vi "Reply.vi"(8 "error in (no error)":errorcluster, 10 "Reply":refnum<class "MSG.lvclass"> caption="Reply (Label superceeded by reply label if provided by \"Message to reply to\")", 11 "Message to Reply to":refnum<class "MSG.lvclass">) -> (0 "error out":errorcluster, 3 "Message":refnum<class "MSG.lvclass">)   [LabVIEW 2011, in "Messenging.lvlib" / "MSG.lvclass"]
uses:
  MSG.lvclass
  ErrorMessage/ErrorMessage.lvclass
  Send/Send.lvclass
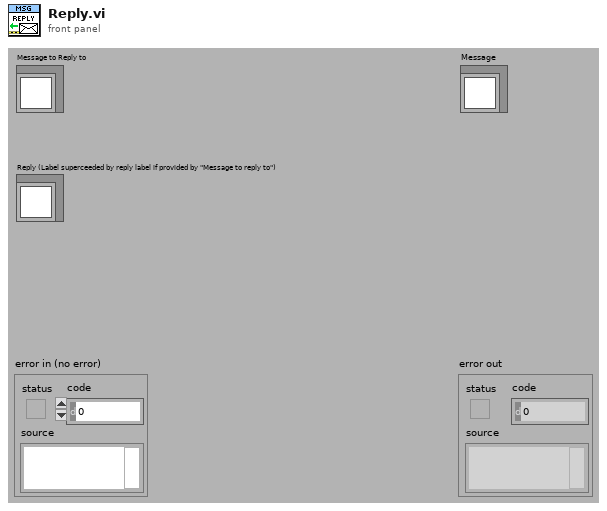
[diagram p1: front panel]
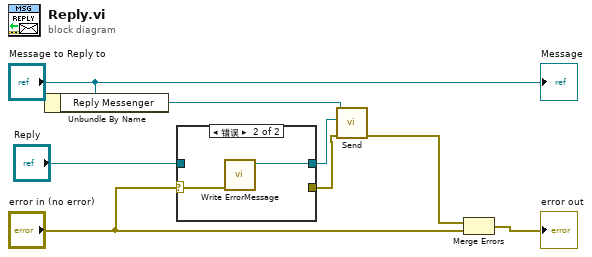
[diagram p0: block diagram]
diagram:
  n1 = Unbundle By Name("Message to Reply to") -> ("Reply Messenger"=w6:refnum<class "Send.lvclass">)
  n2 = case shown="错误" "error in (no error)" {
    selector: "error in (no error)" -> [w9 w11]
    tunnel: [w10 w12] -> w5
    tunnel: "Reply" -> [w10 _]
    tunnel: [w9 _] -> w3
    frame No Error {
    }
    frame Error {
      n3 = call "Write ErrorMessage.vi"("error (to be sent)"=w11) -> ("Message"=w12:refnum<class "ErrorMessage.lvclass">)  [unwired: 2 in, 8 out]
    }
  }
  n4 = call-dynamic "Send.vi"("error in (no error)"=w3, "Message"=w5, "MSR Parent in"=w6) -> ("error out"=w8:errorcluster)  [unwired: 8 out]
  n5 = Merge Errors(w8, "error in (no error)") -> (→"error out":errorcluster)
  "Message" <- "Message to Reply to"
